vi "ramp.vi"(2 "TimeParams":dbl[](array[numeric])=[1.0, 1.0, 1.0, 1.0, 1.0], 3 "Seq":dbl[](array[numeric])=[30.0, 50.0, 60.0, 30.0, 20.0], 5 "T_man":dbl, 7 "manual":i32, 8 "port":i32=1, 10 "reset":bool, 11 "pause":bool=TRUE) -> (0 "T control":dbl, 1 "STEP":i32, 4 "params":i32[](array[numeric]), 6 "T ext":dbl, 9 "T in":dbl)   [LabVIEW 2015]
uses:
  x64/Debug/BERTTA.dll
panel:
  out "Waveform Chart":dynamicdata(graph)
  out "params2":i32
  out "params0":i32
  out "params1":i32
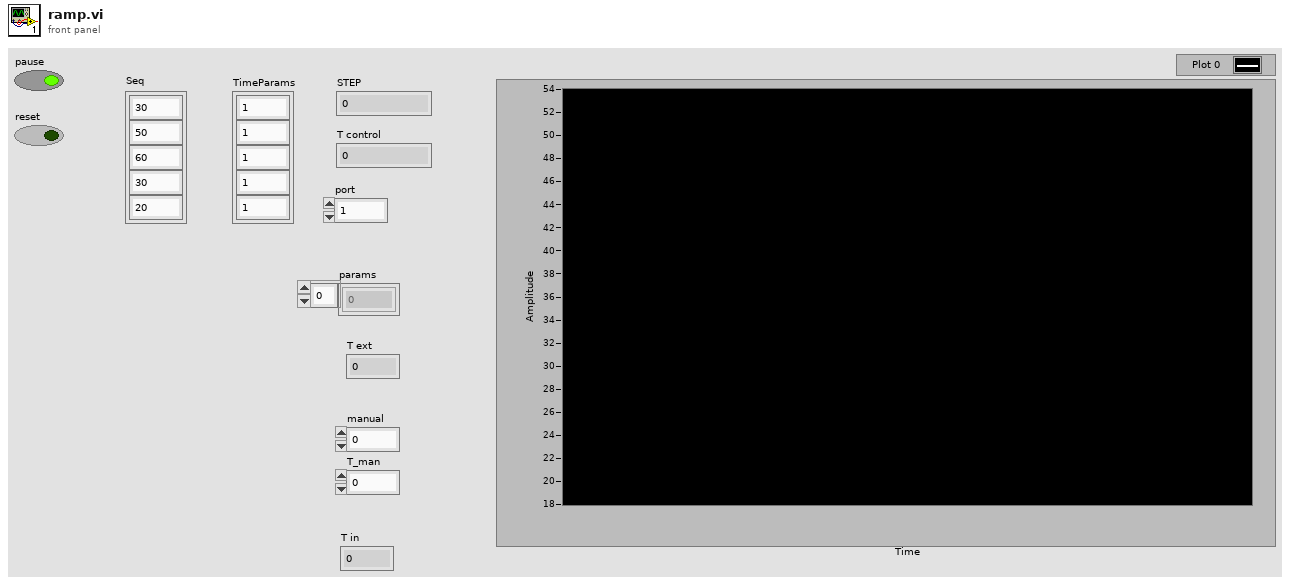
[diagram p1: front panel]
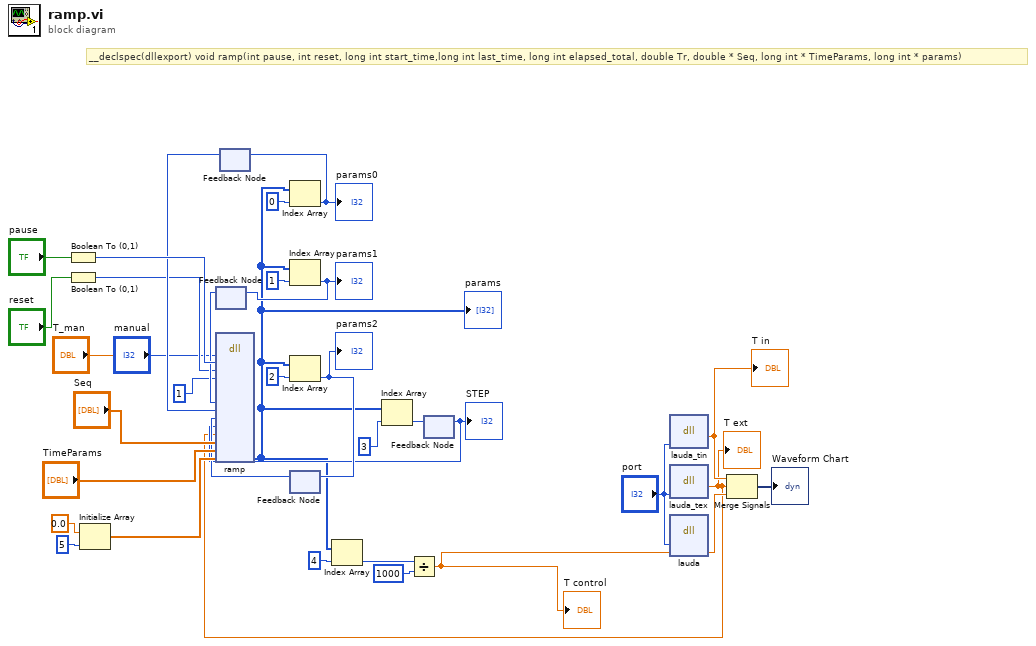
[diagram p0: block diagram]
diagram:
  # "__declspec(dllexport) void ramp(int pause, int reset, long int start_time,long int last_time, long int elapsed_total, double Tr, double * Seq, long int * TimeParams, long int * params)"
  n1 = Boolean To (0,1)(Boolean="pause") -> (0, 1=w27:i16)
  n2 = Boolean To (0,1)(Boolean="reset") -> (0, 1=w21:i16)
  n3 = Initialize Array(0.0 ("element"), 5 ("dimension size")) -> (w34:dbl[])
  n4 = feedback #1() -> (w23:i32)  [unwired: 1 in]
  n5 = feedback #2() -> (w24:i32)  [unwired: 1 in]
  n6 = feedback #3() -> (w18:i32)  [unwired: 1 in]
  n7 = feedback #4() -> (w14:i32)  [unwired: 1 in]
  "STEP" <- w14
  n8 = dll-call lib="C:/Users/shresplab/OneDrive - Kemira Oyj/Documents/Visual Studio 2017/Projects/Bertta/BERTTA/x64/Debug/BERTTA.dll" fn="lauda_tin"("port"="port") -> ("return type"=w11:dbl)  [unwired: 4 in, 2 out]
  "T in" <- w11
  n9 = dll-call lib="C:/Users/shresplab/OneDrive - Kemira Oyj/Documents/Visual Studio 2017/Projects/Bertta/BERTTA/x64/Debug/BERTTA.dll" fn="lauda_tex"("port"="port") -> ("return type"=w6:dbl)  [unwired: 4 in, 2 out]
  "T ext" <- w6
  n10 = dll-call lib="C:/Users/shresplab/OneDrive - Kemira Oyj/Documents/Visual Studio 2017/Projects/Bertta/BERTTA/x64/Debug/BERTTA.dll" fn="ramp"("pause"=w27, "reset"=w21, "grad"=1, "manual"="manual", "T_man"="T_man", "start_time"=w23, "last_time"=w24, "elapsed_total"=w18, "step"=w14, "Tr"=w6, "Seq"="Seq", "TimeParams"="TimeParams", "params"=w34) -> ("params"=w9:i32[])  [unwired: 16 in, 2 out]
  "params" <- w9
  n11 = Index Array(array=w9, index=0) -> (element=w29:i32)
  "params0" <- w29
  n12 = feedback-in #2(w29) -> ()
  n13 = Index Array(array=w9, index=1) -> (element=w28:i32)
  "params1" <- w28
  n14 = feedback-in #1(w28) -> ()
  n15 = Index Array(array=w9, index=2) -> (element=w17:i32)
  "params2" <- w17
  n16 = feedback-in #3(w17) -> ()
  n17 = Index Array(array=w9, index=4) -> (element=w8:i32)
  n18 = Index Array(array=w9, index=3) -> (element=w15:i32)
  n19 = Divide(x=w8, y=1000) -> (x/y=w5:dbl)
  "T control" <- w5
  n20 = feedback-in #4(w15) -> ()
  n21 = dll-call lib="C:/Users/shresplab/OneDrive - Kemira Oyj/Documents/Visual Studio 2017/Projects/Bertta/BERTTA/x64/Debug/BERTTA.dll" fn="lauda"("port"="port", "set_temp"=w5) -> ("set_temp"=w12:dbl)  [unwired: 5 in, 2 out]
  n22 = Merge Signals(w11, w6, w12) -> (→"Waveform Chart":dynamicdata)
